vi "Resistance1.vi"() -> ()   [LabVIEW 2017]
uses:
  <instrlib>/Keithley 6517/Keithley 6517.lvlib
panel:
  in  "Timeout(10000 ms)":u32=10000
  in  "source amplitude (2.0000000E+2) 4":dbl=200.0 format="%.7e"
  out "Measurement":T1 {"Measurement" format="%.6e"}
  in  "LO connecction 2":bool
  in  "Display Resolution (6)":dbl=6.0
  in  "Auto Range Value (2.0000000E+2)":dbl=200.0 format="%.7e"
  in  "Measurement Function (2: Resistance)":i32(ring) items=["Voltage", "Current", "Resistance", "Charge"]
  in  "VISA resource name":refnum<visa-resource-name>
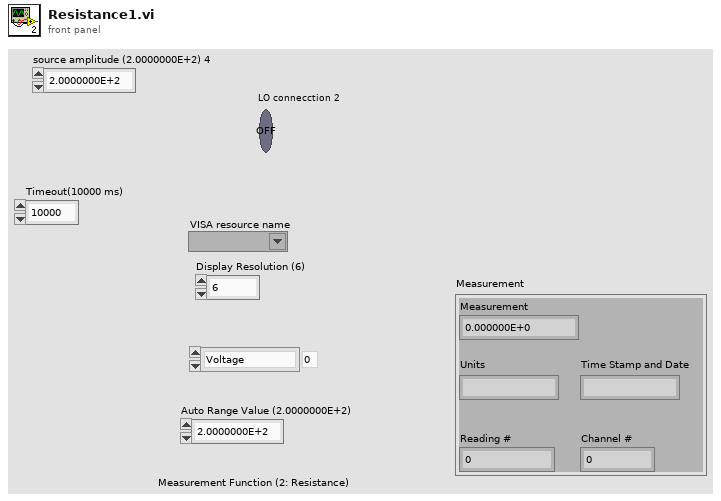
[diagram p1: front panel]
types:
  T1 = cluster{"Measurement":dbl, "Units":string, "Time Stamp and Date":string, "Reading #":dbl, "Channel #":dbl}
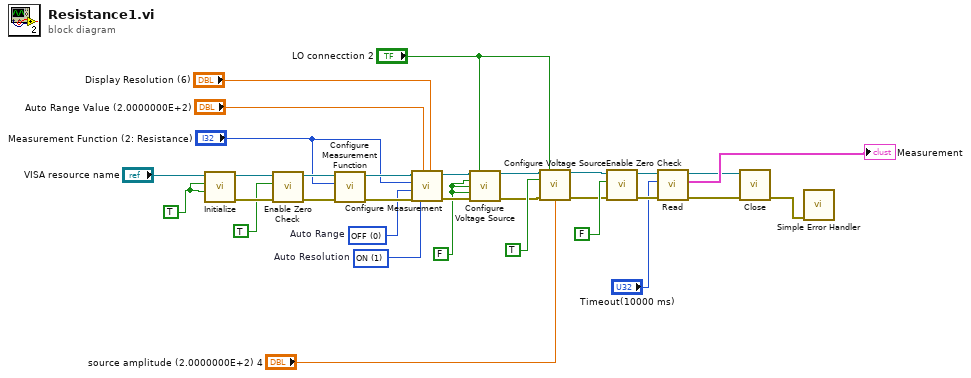
[diagram p0: block diagram]
diagram:
  w8 = FALSE
  w24 = 1 items=["OFF", "ON", "ONCE"]  # Auto Resolution
  w23 = 0 items=["OFF", "ON", "ONCE"]  # Auto Range
  w31 = TRUE
  n1 = call <instrlib>:"Initialize.vi"("Reset (True)"=w31, "ID Query (True)"=w31, "VISA resource name"="VISA resource name") -> ("error out"=w30:errorcluster, "VISA resource name out"=w29:refnum<visa-resource-name>)  [unwired: 7 in]
  n2 = call <instrlib>:"Enable Zero Check.vi"("error in (no error)"=w30, "Enable Zero Check (T: Enable)"=TRUE, "VISA resource name"=w29) -> ("error out"=w27:errorcluster, "VISA resource name out"=w28:refnum<visa-resource-name>)  [unwired: 7 in]
  n3 = call <instrlib>:"Configure Measurement Function.vi"("error in (no error)"=w27, "Measurement Function (0: Voltage)"="Measurement Function (2: Resistance)", "VISA resource name"=w28) -> ("error out"=w25:errorcluster, "VISA resource name out"=w26:refnum<visa-resource-name>)  [unwired: 7 in]
  n4 = call <instrlib>:"Configure Measurement.vi"("Display Resolution (6)"="Display Resolution (6)", "Auto Resolution (1: ON)"=w24, "Auto Range Value (2.0000000E+2)"="Auto Range Value (2.0000000E+2)", "error in (no error)"=w25, "Auto Range (1: ON)"=w23, "Measurement Function (0: Voltage)"="Measurement Function (2: Resistance)", "VISA resource name"=w26) -> ("error out"=w12:errorcluster, "VISA resource name out"=w13:refnum<visa-resource-name>)  [unwired: 3 in]
  n5 = call <instrlib>:"Configure Voltage Source.vi"("VISA resource name"=w13, "Enable LO Connection (F: Disable)"="LO connecction 2", "Enable V-source (F: Disable)"=w8, "Enable Voltage Limit (F: Disable)"=w8, "Enable Resistance Current Limit (F: Disable)"=w8, "error in (no error)"=w12) -> ("VISA resource name out"=w11:refnum<visa-resource-name>, "error out"=w10:errorcluster)  [unwired: 8 in]
  n6 = call <instrlib>:"Configure Voltage Source.vi"("VISA resource name"=w11, "Enable LO Connection (F: Disable)"="LO connecction 2", "Enable V-source (F: Disable)"=TRUE, "error in (no error)"=w10, "V-source Amplitude (0.000000E+0)"="source amplitude (2.0000000E+2) 4") -> ("VISA resource name out"=w16:refnum<visa-resource-name>, "error out"=w15:errorcluster)  [unwired: 9 in]
  n7 = call <instrlib>:"Enable Zero Check.vi"("error in (no error)"=w15, "Enable Zero Check (T: Enable)"=FALSE, "VISA resource name"=w16) -> ("error out"=w6:errorcluster, "VISA resource name out"=w5:refnum<visa-resource-name>)  [unwired: 7 in]
  n8 = call <instrlib>:"Read.vi"("error in (no error)"=w6, "Timeout(10000 ms)"="Timeout(10000 ms)", "VISA resource name"=w5) -> ("error out"=w4:errorcluster, "Measurement"=→"Measurement":T1, "VISA resource name out"=w2:refnum<visa-resource-name>)  [unwired: 6 in]
  n9 = call <instrlib>:"Close.vi"("error in (no error)"=w4, "VISA resource name"=w2) -> ("error out"=w18:errorcluster)  [unwired: 9 in]
  n10 = call <vilib>:"Simple Error Handler.vi"("error in (no error)"=w18) -> ()  [unwired: 4 in, 5 out]
